vi "propeller_horizontal_force_calculation.vi"(6 "acceleration_magnitude":dbl, 9 "drag_magnitude":dbl, 10 "mass":dbl, 11 "reaction":dbl) -> (3 "propeller_horizontal_force":dbl)   [LabVIEW 2018]
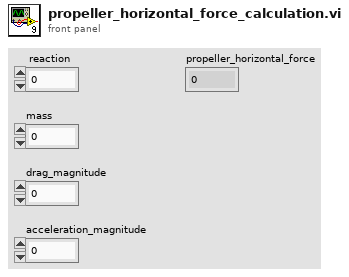
[diagram p1: front panel]
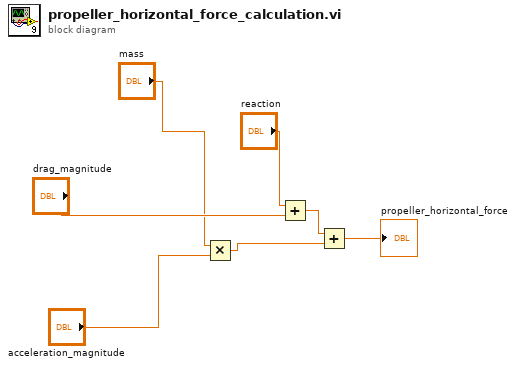
[diagram p0: block diagram]
diagram:
  n1 = Multiply(x="mass", y="acceleration_magnitude") -> (x*y=w4:dbl)
  n2 = Add(x="reaction", y="drag_magnitude") -> (x+y=w3:dbl)
  n3 = Add(x=w3, y=w4) -> (x+y=→"propeller_horizontal_force":dbl)
